vi "Initialization.vi"(8 "Error In":errorcluster) -> (0 "Error Out":errorcluster)   [LabVIEW 2019]
uses:
  WSCbot_V3_Toolkit.lvlibp/WSCBOTV3_Toolkit/IO/LowLevel/PulseCounter.ctl
  WSCbot_V3_Toolkit.lvlibp/WSCBOTV3_Toolkit/IO/LowLevel/IO_Chanel_DIO.ctl
  WSCbot_V3_Toolkit.lvlibp
panel:
  out "Hight":i32
  out "Angle_index":i32
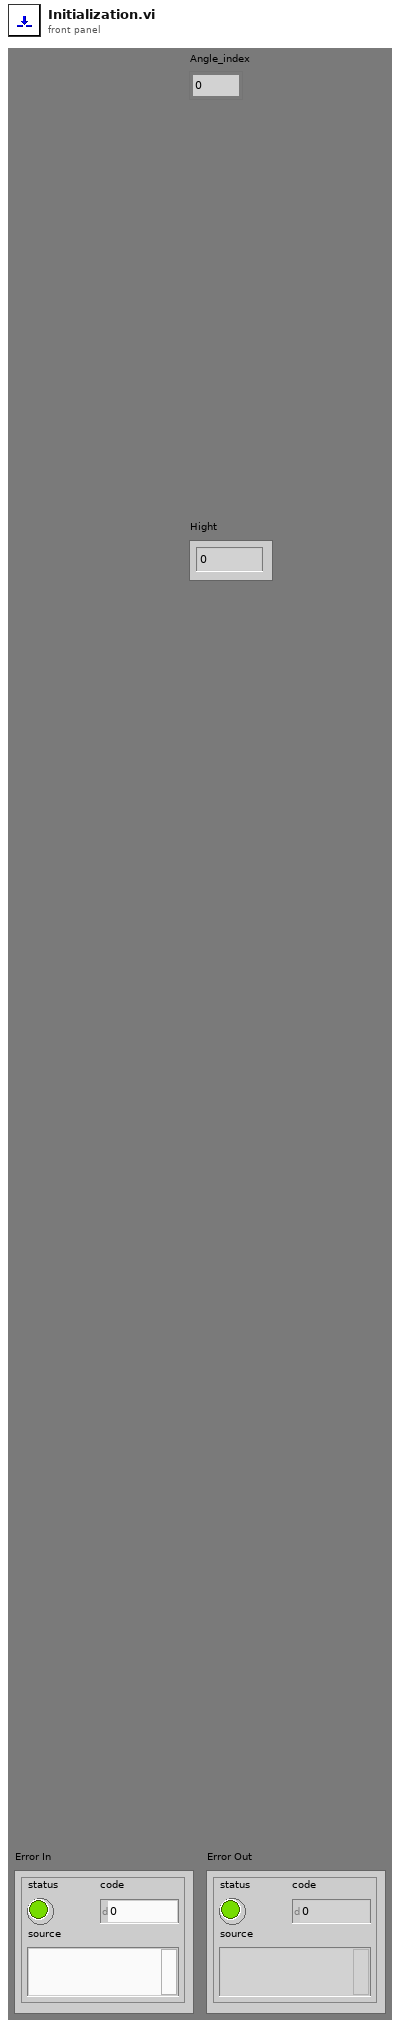
[diagram p1: front panel]
types:
  T1 = typedef "WSCbot_V3_Toolkit.lvlibp/PulseCounter.ctl" = enum16{"CH1", "CH2", "CH3", "CH4", "CH5"}
  T2 = typedef "WSCbot_V3_Toolkit.lvlibp/IO_Chanel_DIO.ctl" = enum16{"A/DIO9", "A/DIO10", "C/DIO0", "C/DIO1", "C/DIO2", "C/DIO3", "C/DIO4", "C/DIO5", "C/DIO6"}
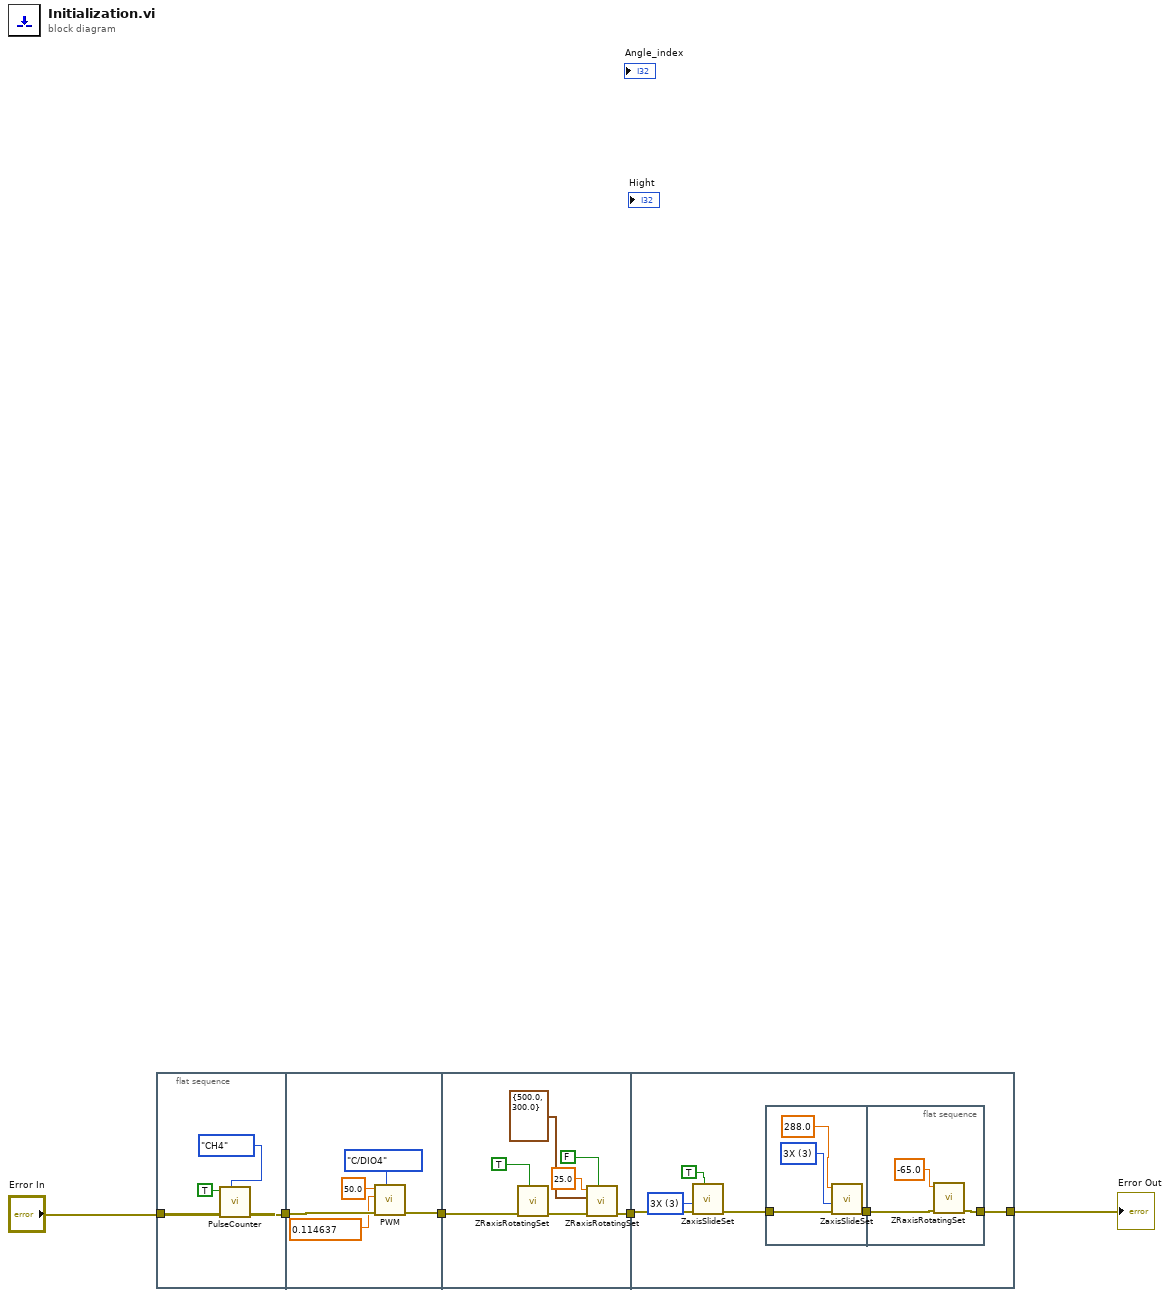
[diagram p0: block diagram]
diagram:
  n1 = flat-sequence {
    tunnel: "Error In" -> [w7]
    tunnel: [w6] -> w2
    tunnel: [w13] -> w5
    tunnel: w2 -> [w14]
    tunnel: [w16] -> w4
    tunnel: w5 -> [w15]
    tunnel: w4 -> [w25]
    tunnel: [w23] -> w1
    frame #0 {
      n2 = call "PulseCounter.vi"("PulseCounterChanel"=PulseCounter."CH4", "error in"=w7, "Reset"=TRUE) -> ("error out"=w6:errorcluster)  [unwired: 7 in, 1 out]
    }
    frame #1 {
      n3 = call "PWM.vi"("IO_Chanel"=IO_Chanel_DIO."C/DIO4", "error in"=w14, "DutyCycle"=0.114637, "Frequency(Hz)"=50.0) -> ("error out"=w13:errorcluster)  [unwired: 7 in]
    }
    frame #2 {
      n4 = call "ZRaxisRotatingSet.vi"("Reset"=TRUE, "error in"=w15) -> ("error out"=w20:errorcluster)  [unwired: 8 in, 1 out]
      n5 = call "ZRaxisRotatingSet.vi"("Reset"=FALSE, "error in"=w20, "Velocity(deg/s)&ACC(deg/ss)"=cluster{"Velocity(cm/s)":dbl, "ACC(cm/ss)":dbl} {"Velocity(cm/s)"=500.0, "ACC(cm/ss)"=300.0}, "TargetHight(deg)"=25.0) -> ("error out"=w16:errorcluster)  [unwired: 6 in, 1 out]
    }
    frame #3 {
      w26 = u16 3 items=["0X", "1X", "2X", "3X"] ("findHomeVel (times)")
      n6 = call "ZaxisSlideSet.vi"("Reset"=TRUE, "error in"=w25, "findHomeVel (times)"=w26) -> ("error out"=w22:errorcluster)  [unwired: 7 in, 1 out]
      n7 = flat-sequence {
        tunnel: [w31] -> w24
        tunnel: w22 -> [w28]
        tunnel: w24 -> [w34]
        tunnel: [w32] -> w23
        frame #0 {
          w30 = u16 3 items=["0X", "1X", "2X", "3X"] ("findHomeVel (times)")
          n8 = call "ZaxisSlideSet.vi"("error in"=w28, "findHomeVel (times)"=w30, "TargetABSHight(mm)"=288.0) -> ("error out"=w31:errorcluster)  [unwired: 7 in, 1 out]
        }
        frame #1 {
          n9 = call "ZRaxisRotatingSet.vi"("error in"=w34, "TargetHight(deg)"=-65.0) -> ("error out"=w32:errorcluster)  [unwired: 8 in, 1 out]
        }
      }
    }
  }
  "Error Out" <- w1
